vi "Var_señales.vi"() -> ()   [LabVIEW 2018]
panel:
  in  "Var_V":sgl
  in  "Var_Frec":sgl
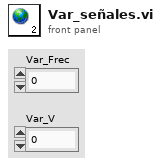
[diagram p1: front panel]
diagram:
